vi "Read Proportional.vi"(8 "error in (no error)":errorcluster, 11 "Lakeshore Gaussmeter in":refnum<class "Lakeshore Gaussmeter.lvclass">) -> (0 "error out":errorcluster, 2 "Proportional":dbl, 3 "Lakeshore Gaussmeter out":refnum<class "Lakeshore Gaussmeter.lvclass">)   [LabVIEW 2023, in "Lakeshore Gaussmeter.lvclass"]
uses:
  Lakeshore Gaussmeter.lvclass
  Lakeshore Gaussmeter.lvclass/Lakeshore Gaussmeter.ctl
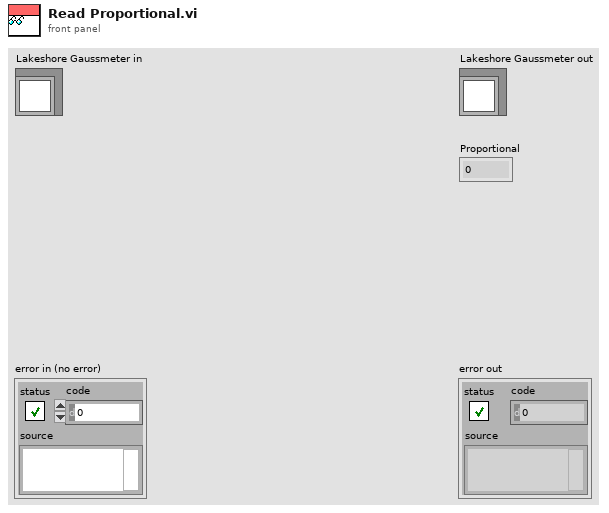
[diagram p1: front panel]
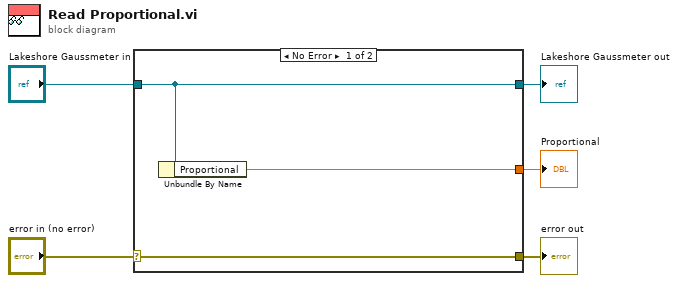
[diagram p0: block diagram]
diagram:
  n1 = case shown="No Error" "error in (no error)" {
    selector: "error in (no error)" -> [w8 w9]
    tunnel: [w8 w9] -> w4
    tunnel: [w7 w10] -> w2
    tunnel: "Lakeshore Gaussmeter in" -> [w7 w10]
    tunnel: [w6 _] -> w1
    frame No Error {
      n2 = Unbundle By Name(w7) -> ("Proportional"=w6:dbl)
    }
    frame Error {
    }
  }
  "error out" <- w4
  "Lakeshore Gaussmeter out" <- w2
  "Proportional" <- w1
